vi "add datafile(SubVI).vi"(10 "字符串":string) -> (1 "ok or cancel":bool=TRUE, 2 "连接的字符串":string)   [LabVIEW 2019, in "Add Seq.lvlib"]
uses:
  Add Seq.lvlib
panel:
  in  "cancel":bool
  in  "ok":bool
  in  "operation(0:open)":T1(ring)=enum."create"
  in  "path":path
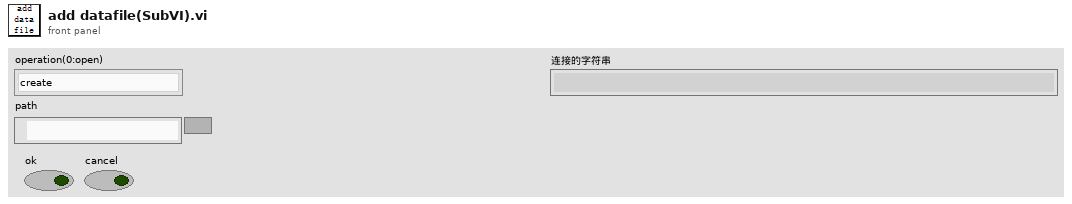
[diagram p1: front panel]
types:
  T1 = enum16{"open", "replace", "create", "open or create", "replace or create"}
  T2 = enum16{"open", "replace", "create", "open or create", "replace or create", "replace or create with confirmation"}
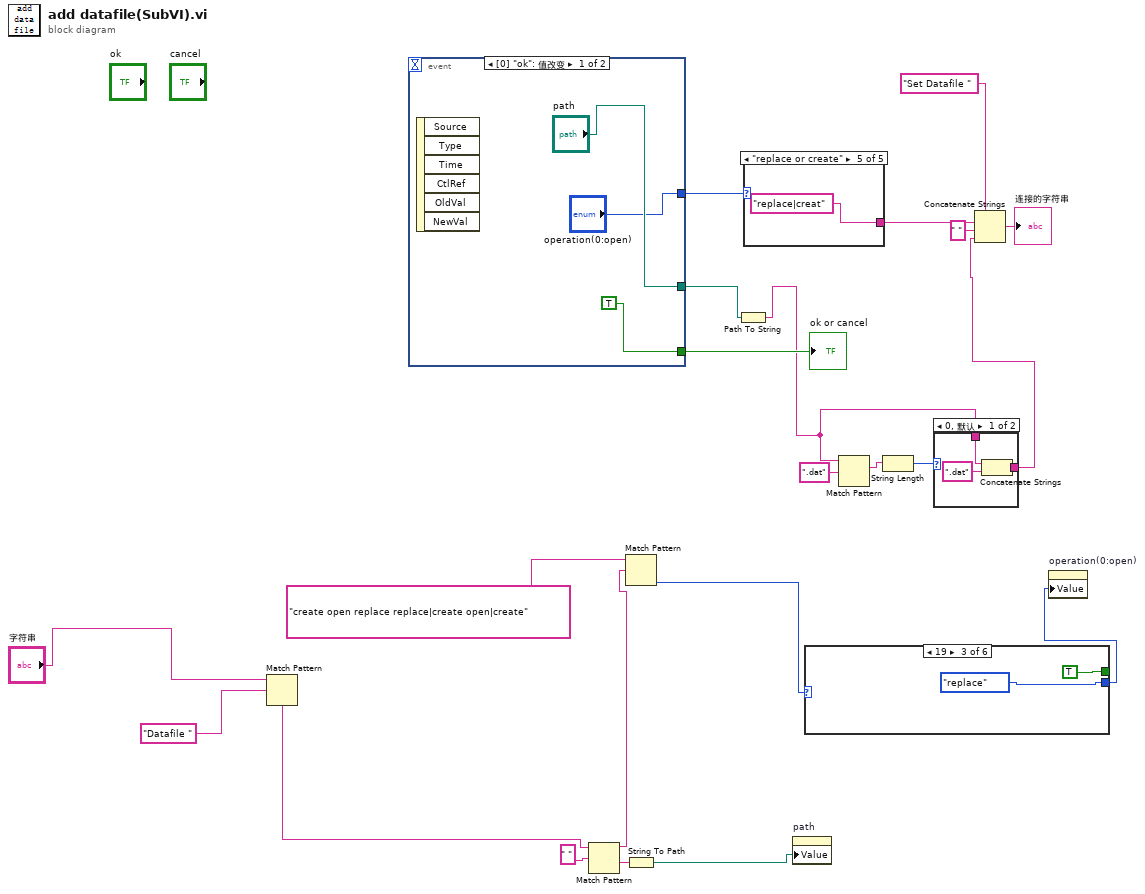
[diagram p0: block diagram]
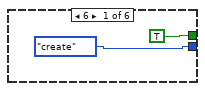
[diagram p2: hidden frame]
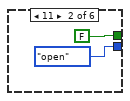
[diagram p3: hidden frame]
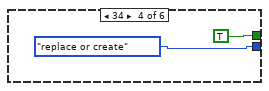
[diagram p4: hidden frame]
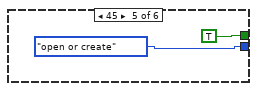
[diagram p5: hidden frame]
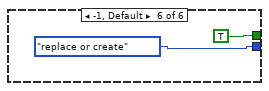
[diagram p6: hidden frame]
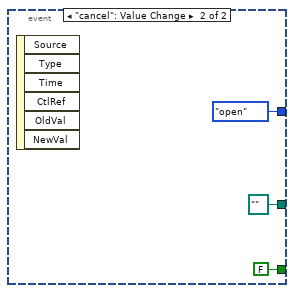
[diagram p8: hidden frame]
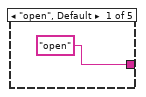
[diagram p9: hidden frame]
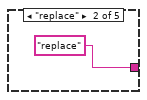
[diagram p10: hidden frame]
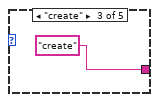
[diagram p11: hidden frame]
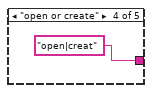
[diagram p12: hidden frame]
diagram:
  n1 = Match Pattern(string="字符串", regular expression="Datafile " ("正则表达式")) -> (after substring=w9:string)  [unwired: 1 in, 3 out]
  n2 = event shown="[0] \"ok\": 值改变" {
    selector: _ -> [_ _]
    dyn-events: _ -> [_ _]
    timeout: _ -> [_ _]
    tunnel: ["path" path "" ("path")] -> w16
    tunnel: ["operation(0:open)" T1."open" ("operation(0:open)")] -> w21
    tunnel: [TRUE FALSE] -> w17
    event "ok": Value Change {
      n3 = event-data() -> ()  [unwired: 1 in, 6 out]
    }
    event "cancel": Value Change {
      n4 = event-data() -> ()  [unwired: 1 in, 6 out]
    }
  }
  "ok or cancel" <- w17
  n5 = Match Pattern(string=w9, regular expression=" " ("正则表达式")) -> (before substring=w7:string, after substring=w5:string)  [unwired: 1 in, 2 out]
  n6 = Match Pattern(string="create open replace replace|create open|create" ("字符串"), regular expression=w7) -> (offset past match=w4:i32)  [unwired: 1 in, 3 out]
  n7 = String To Path(string=w5) -> (path=w2:path)
  n8 = Path To String(path=w16) -> (string=w12:string)
  n9 = case shown="\"replace or create\"" w21 {
    tunnel: ["open" "replace" "create" "open|creat" "replace|creat"] -> w20
    frame "open", Default {
    }
    frame "replace" {
    }
    frame "create" {
    }
    frame "open or create" {
    }
    frame "replace or create" {
    }
  }
  n10 = property on="path" class="Path"("Value"=w2) -> ()  [unwired: 2 in, 2 out]
  n11 = case shown="19" w4 {
    tunnel: [T2."create" ("操作(0:open)") T2."open" ("操作(0:open)") T2."replace" ("操作(0:open)") T2."replace or create" ("操作(0:open)") T2."open or create" ("操作(0:open)") T2."replace or create" ("操作(0:open)")] -> w3
    tunnel: [TRUE FALSE TRUE TRUE TRUE TRUE] -> _
    frame 6 {
    }
    frame 11 {
    }
    frame 19 {
    }
    frame 34 {
    }
    frame 45 {
    }
    frame -1, Default {
    }
  }
  n12 = Match Pattern(string=w12, regular expression=".dat" ("正则表达式")) -> (match substring=w14:string)  [unwired: 1 in, 3 out]
  n13 = String Length(string=w14) -> (length=w13:i32)
  n14 = case shown="0, 默认" w13 {
    tunnel: w12 -> [w48 w49]
    tunnel: [w46 w49] -> w11
    frame 0, Default {
      n15 = Concatenate Strings(w48, ".dat" ("字符串")) -> (w46:string)
    }
    frame 4 {
    }
  }
  n16 = Concatenate Strings("Set Datafile " ("字符串"), w20, " " ("字符串"), w11) -> (→"连接的字符串":string)
  n17 = property on="operation(0:open)" class="Enum (严格)"("Value"=w3) -> ()  [unwired: 2 in, 2 out]
